vi "paneValue.vi"() -> ()   [LabVIEW 2017]
uses:
  <vilib>/Utility/miscctls.llb/LVRectTypeDef.ctl
  user32.dll
panel:
  out "Front Panel Window:Panel Bounds":T1
  out "POINT":i32[](array[numeric])
  out "Position:Left 2":i32
  out "Position:Top 2":i32
  out "Position:Top":i32
  out "Position:Left":i32
  in  "Model Selection:-":string(combo)
  in  "stop":bool
  in  "BARCODE STATION 3":string caption="QR CODE :-"
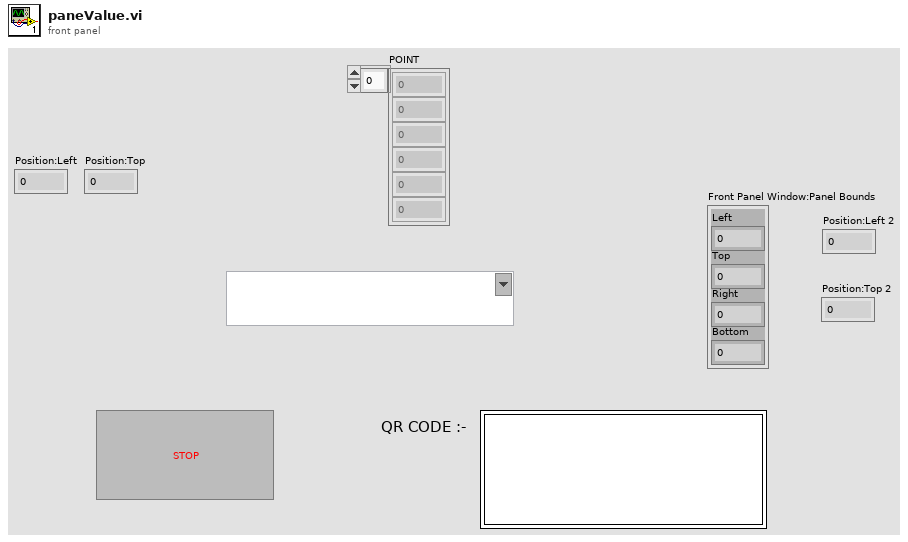
[diagram p1: front panel]
types:
  T1 = typedef "LVRectTypeDef.ctl" = cluster{"Left":i16, "Top":i16, "Right":i16, "Bottom":i16}
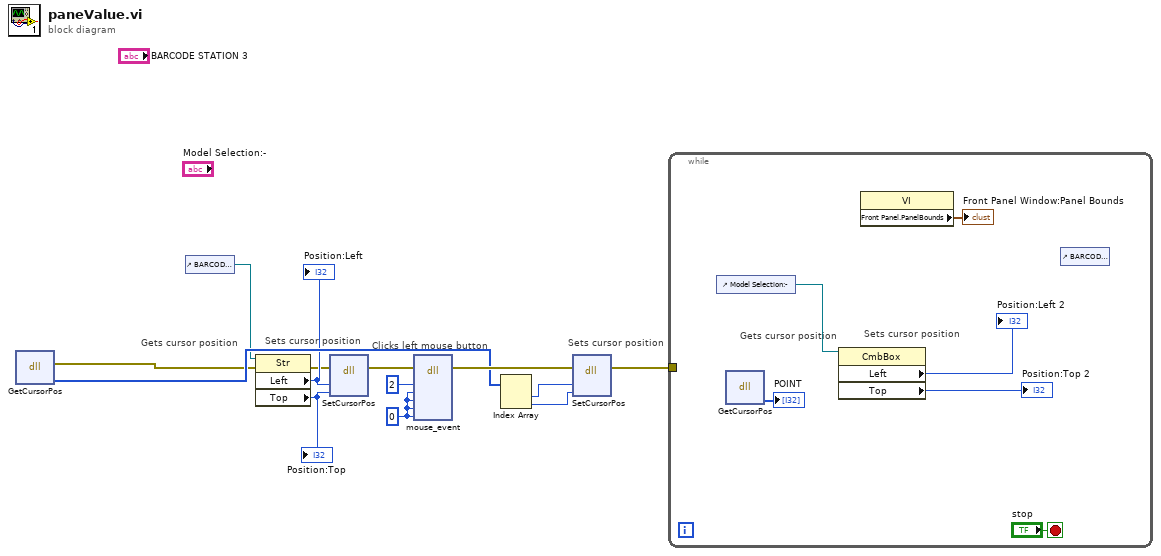
[diagram p0: block diagram]
diagram:
  w13 = u32 0 ("dy")
  # "Sets cursor position"
  # "Gets cursor position"
  # "Clicks left mouse button"
  # "Sets cursor position"
  n1 = dll-call lib="User32.dll" fn="GetCursorPos" ("Move mouse to new pos")() -> (error out=w6:errorcluster, "POINT"=w9:i32[])  [unwired: 5 in, 1 out]
  n2 = control-ref of="BARCODE STATION 3"() -> (w2:refnum<vi>)
  n3 = property on="Property Node" class="Str"(reference=w2, error in=w6) -> (error out=w5:errorcluster, "Left"=w8:i32, "Top"=w7:i32)  [unwired: 1 out]
  "Position:Left" <- w8
  "Position:Top" <- w7
  n4 = dll-call lib="User32.dll" fn="SetCursorPos" ("Move mouse to new pos")(error in=w5, "dx"=w8, "dy"=w7) -> (error out=w10:errorcluster)  [unwired: 5 in, 1 out]
  n5 = dll-call lib="user32.dll" fn="mouse_event"(error in=w10, "dwFlags"=u32 2, "dx"=w13, "dy"=w13, "dwData"=w13, "dwExtraInfo"=w13) -> (error out=w12:errorcluster)  [unwired: 8 in, 1 out]
  n6 = Index Array(array=w9) -> (element #1=w3:i32, element #2=w4:i32)  [unwired: 2 in]
  n7 = dll-call lib="User32.dll" fn="SetCursorPos" ("Move mouse to new pos")(error in=w12, "dx"=w3, "dy"=w4) -> (error out=w1:errorcluster)  [unwired: 5 in, 1 out]
  n8 = while {
    tunnel: w1 -> [_]
    stop <- "stop" stop-if-true
    # "Gets cursor position"
    # "Sets cursor position"
    n9 = control-ref of="Model Selection:-"() -> (w15:refnum<vi>)
    n10 = dll-call lib="User32.dll" fn="GetCursorPos" ("Move mouse to new pos")() -> ("POINT"=→"POINT":i32[])  [unwired: 5 in, 2 out]
    n11 = property on="Property Node" class="CmbBox"(reference=w15) -> ("Left"=→"Position:Left 2":i32, "Top"=→"Position:Top 2":i32)  [unwired: 1 in, 2 out]
    n12 = property class="VI"() -> ("Front Panel.PanelBounds"=→"Front Panel Window:Panel Bounds":T1)  [unwired: 2 in, 2 out]
    n13 = control-ref of="BARCODE STATION 3"() -> ()  [unwired: 1 out]
  }
